vi "BLMultiplotPrepare.vi"(6 "HeightAxisBounds":T1, 7 "ProfileFilename":string, 8 "NormaliseHeight?":bool, 9 "YaxisMapping":enum8{"Lin", "Log"}(ring), 10 "jitterFraction":dbl) -> (3 "gnuplotOut":string)   [LabVIEW 2014]
uses:
  minAndMax.ctl
  AutoManualNumber.ctl
  margins.ctl
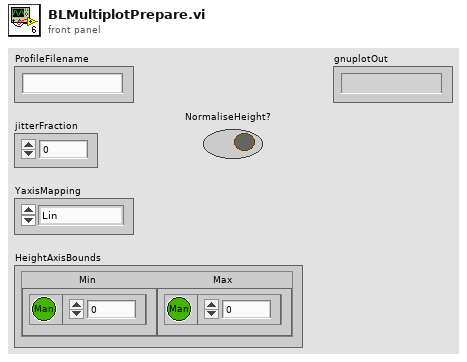
[diagram p1: front panel]
types:
  T1 = typedef "minAndMax.ctl" = cluster{"Min":T2, "Max":T2}
  T2 = typedef "AutoManualNumber.ctl" = cluster{"Auto":bool, "Value":dbl}
  T3 = typedef "margins.ctl" = cluster{"Top":dbl, "Bottom":dbl, "Left":dbl, "Right":dbl}
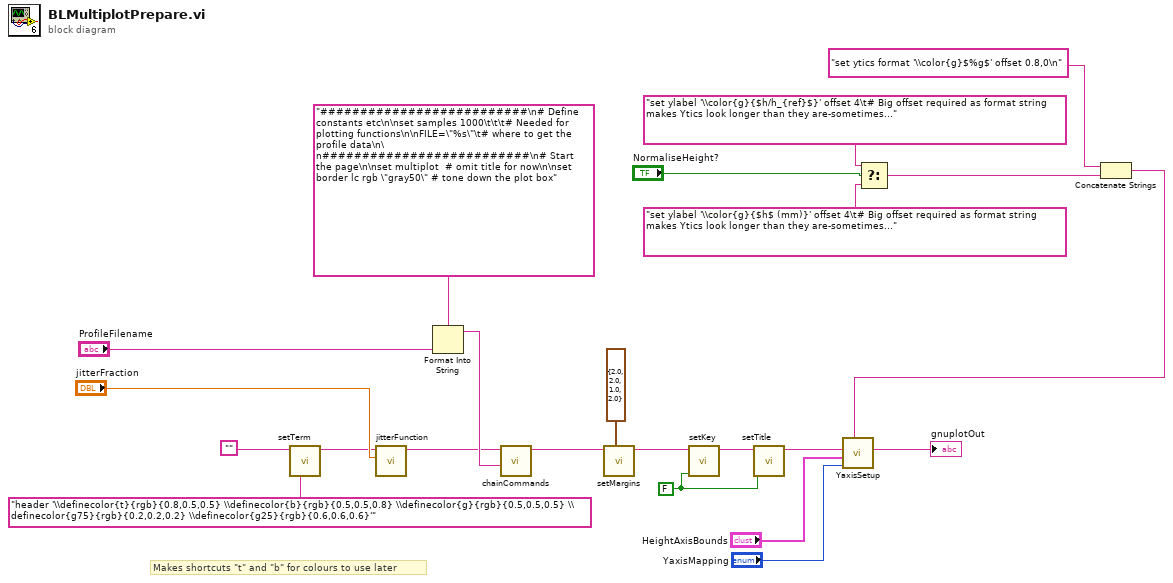
[diagram p0: block diagram]
diagram:
  w18 = FALSE ("Set?")
  # "Makes shortcuts \"t\" and \"b\" for colours to use later"
  n1 = call "setTerm.vi"("Additional Terminal Options"="header '\\definecolor{t}{rgb}{0.8,0.5,0.5} \\definecolor{b}{rgb}{0.5,0.5,0.8} \\definecolor{g}{rgb}{0.5,0.5,0.5} \\definecolor{g75}{rgb}{0.2,0.2,0.2} \\definecolor{g25}{rgb}{0.6,0.6,0.6}'", "String in"="") -> ("String out"=w8:string)  [unwired: 8 in, 1 out]
  n2 = call "jitterFunction.vi"("jitterFraction"="jitterFraction", "String in"=w8) -> ("String out"=w13:string)  [unwired: 8 in, 1 out]
  n3 = Format Into String(format string="##########################\n# Define constants etc\n\nset samples 1000\t\t\t# Needed for plotting functions\n\nFILE=\"%s\"\t# where to get the profile data\n\n##########################\n# Start the page\n\nset multiplot  # omit title for now\n\nset border lc rgb \"gray50\" # tone down the plot box" ("Command"), "ProfileFilename") -> (resulting string=w16:string)  [unwired: 2 in, 1 out]
  n4 = call "chainCommands.vi"("Command"=w16, "StringIn"=w13) -> ("StringOut"=w14:string)  [unwired: 9 in]
  n5 = call "setMargins.vi"("Margins"=T3 {"Top"=2.0, "Bottom"=2.0, "Left"=1.0, "Right"=2.0}, "String in"=w14) -> ("String out"=w11:string)  [unwired: 8 in, 1 out]
  n6 = call "setKey.vi"("Set?"=w18, "String in"=w11) -> ("String out"=w12:string)  [unwired: 8 in, 1 out]
  n7 = call "setTitle.vi"("Set?"=w18, "String in"=w12) -> ("String out"=w19:string)  [unwired: 8 in, 1 out]
  n8 = Select(t="set ylabel '\\color{g}{$h/h_{ref}$}' offset 4\t# Big offset required as format string makes Ytics look longer than they are-sometimes..." ("Post-setup overrides"), s="NormaliseHeight?", f="set ylabel '\\color{g}{$h$ (mm)}' offset 4\t# Big offset required as format string makes Ytics look longer than they are-sometimes..." ("Post-setup overrides")) -> (s? t:f=w3:string)
  n9 = Concatenate Strings("set ytics format '\\color{g}$%g$' offset 0.8,0\n" ("Post-setup overrides"), w3) -> (w2:string)
  n10 = call "YaxisSetup.vi"("Post-setup overrides"=w2, "Mapping"="YaxisMapping", "HeightAxisBounds"="HeightAxisBounds", "gnuplotIn"=w19) -> ("gnuplotOut"=→"gnuplotOut":string)  [unwired: 7 in]
